vi "pass_buoys_details.vi"(0 "Mission in":refnum<class "Mission.lvclass">, 11 "error in (no error)":errorcluster) -> (4 "Mission out":refnum<class "Mission.lvclass">, 6 "Buoy Pass 1":T1 {"North" format="%#_10f"; "East" format="%#_8f"}, 8 "Buoy Pass 2":T1 {"North" format="%#_10f"; "East" format="%#_8f"}, 15 "error out":errorcluster)   [LabVIEW 2011, in "Mission.lvclass"]
uses:
  Mission.lvclass
  2 Typedefs/UTM Location.ctl
  Mission.lvclass/Mission.ctl
panel:
  out "String":string
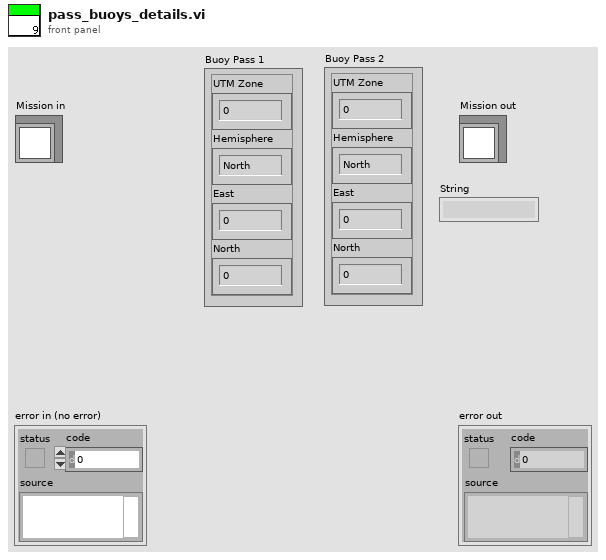
[diagram p1: front panel]
types:
  T1 = typedef "UTM Location.ctl" = cluster{"UTM Zone":dbl, "Hemisphere":enum16{"North", "South"}, "East":dbl, "North":dbl}
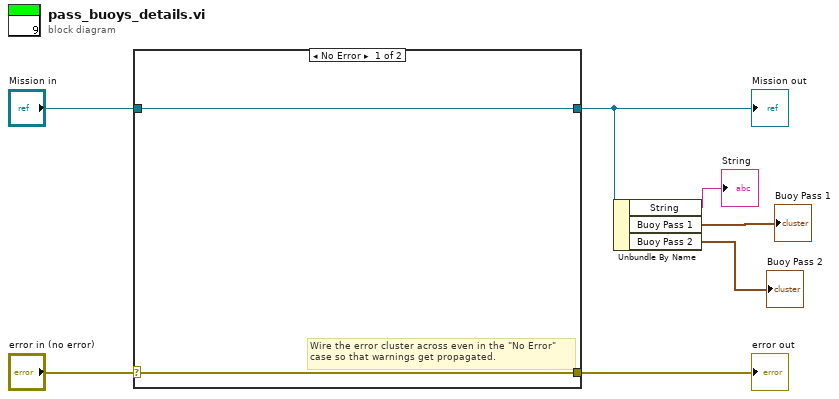
[diagram p0: block diagram]
diagram:
  n1 = case shown="No Error" "error in (no error)" {
    selector: "error in (no error)" -> [w8 w11]
    tunnel: [w8 w11] -> w6
    tunnel: [w9 w10] -> w4
    tunnel: "Mission in" -> [w9 w10]
    frame No Error {
      # "Wire the error cluster across even in the \"No Error\"\ncase so that warnings get propagated."
    }
    frame Error {
    }
  }
  "error out" <- w6
  "Mission out" <- w4
  n2 = Unbundle By Name(w4) -> ("String"=→"String":string, "Buoy Pass 1"=→"Buoy Pass 1":T1, "Buoy Pass 2"=→"Buoy Pass 2":T1)
